vi "LinearSystemId_Elevator_Pack_Model_Params.vi"(5 "DCMOTOR_TYPES":T2, 7 "Num Motors":i32, 9 "Gearing":dbl, 10 "mass_Kg":dbl, 11 "WinchRadius_Meters":dbl) -> (3 "ElevatorSim_Model _Params":T1 {"Gearing" format="%#_13g"; "mass_Kg" format="%#_13g"; "WinchRadias_Meters" format="%#_13g"})   [LabVIEW 2019, in "Trajectory_Library.lvlib"]
uses:
  Trajectory_Library.lvlib
  Enum/DCMOTOR_TYPES_ENUM.ctl
  TypeDef/LINEAR_SYSTEM_ID_ELEVATOR_MODEL.CTL
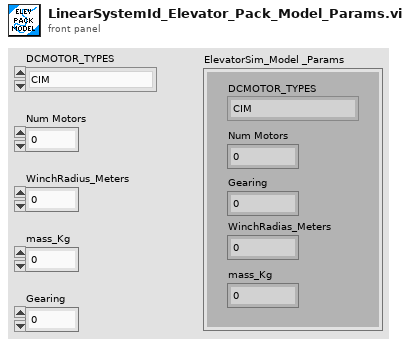
[diagram p1: front panel]
types:
  T1 = typedef "Trajectory_Library.lvlib/LINEAR_SYSTEM_ID_ELEVATOR_MODEL.CTL" = cluster{"DCMOTOR_TYPES":T2, "Num Motors":i32, "WinchRadias_Meters":dbl, "mass_Kg":dbl, "Gearing":dbl}
  T2 = typedef "Trajectory_Library.lvlib/DCMOTOR_TYPES_ENUM.ctl" = enum16{"CIM", "AndyMark 9015", "Andy Mark RS 775 125", "Bag", "BaneBots RS 550", "BaneBots RS 775", "Falcon 500", "Mini CIM", "NEO", "NEO 550", "Romi BuiltIn", "Vex 775 Pro", "Snow Blower AM 2235A", "Bosch Seat AM 3493"}
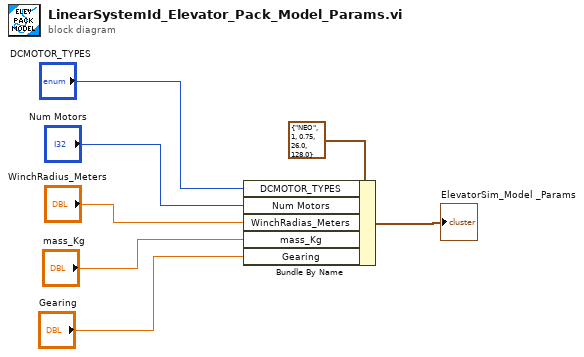
[diagram p0: block diagram]
diagram:
  n1 = Bundle By Name(cluster=T1 {"DCMOTOR_TYPES"=enum."NEO", "Num Motors"=1, "WinchRadias_Meters"=0.75, "mass_Kg"=26.0, "Gearing"=128.0} ("ElevatorSim_Model _Params"), "DCMOTOR_TYPES"="DCMOTOR_TYPES", "Num Motors"="Num Motors", "WinchRadias_Meters"="WinchRadius_Meters", "mass_Kg"="mass_Kg", "Gearing"="Gearing") -> (→"ElevatorSim_Model _Params":T1)
